vi "Move XYZ.vi"(0 "ASI stage":T1, 5 "x":dbl, 7 "y":dbl, 9 "z":dbl, 11 "error in (no error)":errorcluster) -> (15 "error out":errorcluster)   [LabVIEW 2010]
uses:
  stage properties.ctl
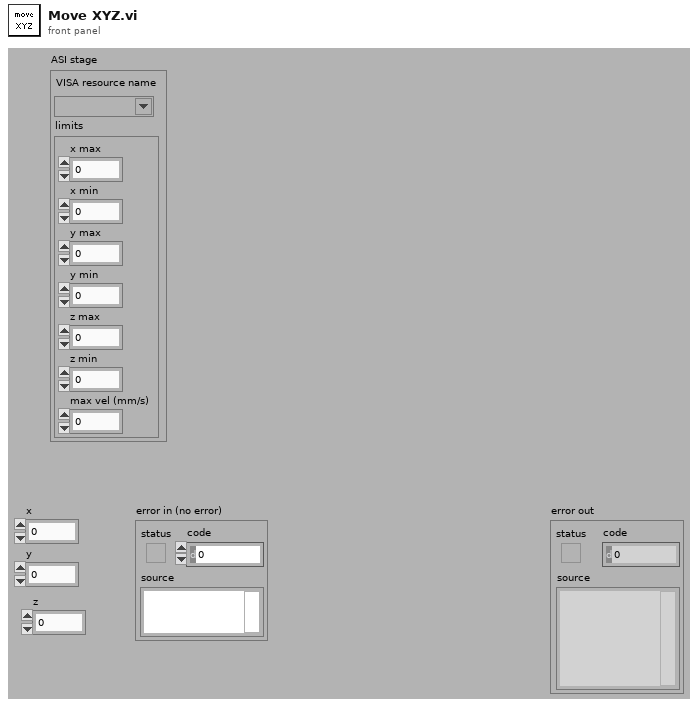
[diagram p1: front panel]
types:
  T1 = typedef "stage properties.ctl" = cluster{"VISA resource name":refnum<visa-resource-name>, "limits":cluster{"x max":dbl, "x min":dbl, "y max":dbl, "y min":dbl, "z max":dbl, "z min":dbl, "max vel (mm/s)":dbl}}
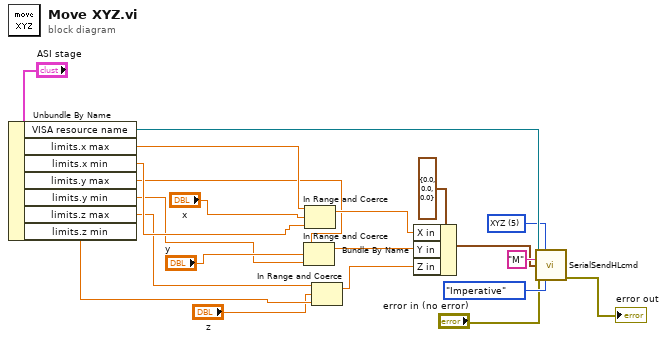
[diagram p0: block diagram]
diagram:
  w19 = u16 5 items=["No axis", "X", "Y", "Z", "XY", "XYZ"] ("Axis configuration")
  n1 = Unbundle By Name("ASI stage") -> ("VISA resource name"=w20:refnum<visa-resource-name>, "limits.x max"=w14:dbl, "limits.x min"=w7:dbl, "limits.y max"=w6:dbl, "limits.y min"=w5:dbl, "limits.z max"=w4:dbl, "limits.z min"=w3:dbl)
  n2 = In Range and Coerce(upper limit=w6, x="y", lower limit=w5) -> (coerced(x)=w11:dbl)  [unwired: 1 out]
  n3 = In Range and Coerce(upper limit=w14, x="x", lower limit=w7) -> (coerced(x)=w10:dbl)  [unwired: 1 out]
  n4 = In Range and Coerce(upper limit=w4, x="z", lower limit=w3) -> (coerced(x)=w1:dbl)  [unwired: 1 out]
  n5 = Bundle By Name(cluster=cluster{"X in":dbl, "Y in":dbl, "Z in":dbl} {"X in"=0.0, "Y in"=0.0, "Z in"=0.0} ("data in"), "X in"=w10, "Y in"=w11, "Z in"=w1) -> (w9:cluster{"X in":dbl, "Y in":dbl, "Z in":dbl})
  n6 = call "SerialSendHLcmd.vi"("VISA resource name"=w20, "Axis configuration"=w19, "Command"="M", "data in"=w9, "error in (no error)"="error in (no error)", "Command type"=enum16{"Query", "Where", "Imperative", "DU Y"}."Imperative") -> ("error out"=→"error out":errorcluster)  [unwired: 7 in, 2 out]
